vi "Repack Pixels_Pixel Bus to FIFO U1x8.vi"(10 "Input Valid":bool=TRUE, 11 "Pixel Bus In":T1={"Pixel Data"=[FALSE, FALSE, FALSE, FALSE, FALSE, FALSE, FALSE, FALSE], "DV"=[FALSE, FALSE, FALSE, FALSE, FALSE, FALSE, FALSE, FALSE], "EOL"=FALSE, "EOI"=FALSE, "Data Type"=enum."U1 x 8"}) -> (2 "Output Valid":bool, 3 "output array":bool[](array[boolean]))   [LabVIEW 2017, in "NI_VDM_FPGA_Basics.lvlib"]
uses:
  <vilib>/visionFPGA/NI_VDM_FPGA_Basics.lvlib
  <vilib>/visionFPGA/Controls/IMAQ FPGA Pixel Bus u1x8.ctl
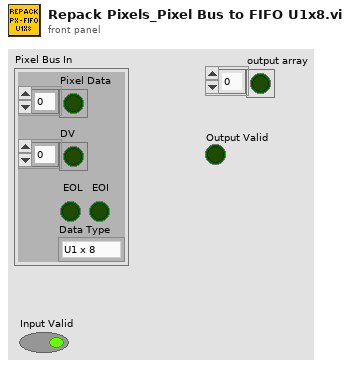
[diagram p1: front panel]
types:
  T1 = typedef "IMAQ FPGA Pixel Bus u1x8.ctl" = cluster{"Pixel Data":bool[], "DV":bool[], "EOL":bool, "EOI":bool, "Data Type":enum16{"U1 x 8"}}
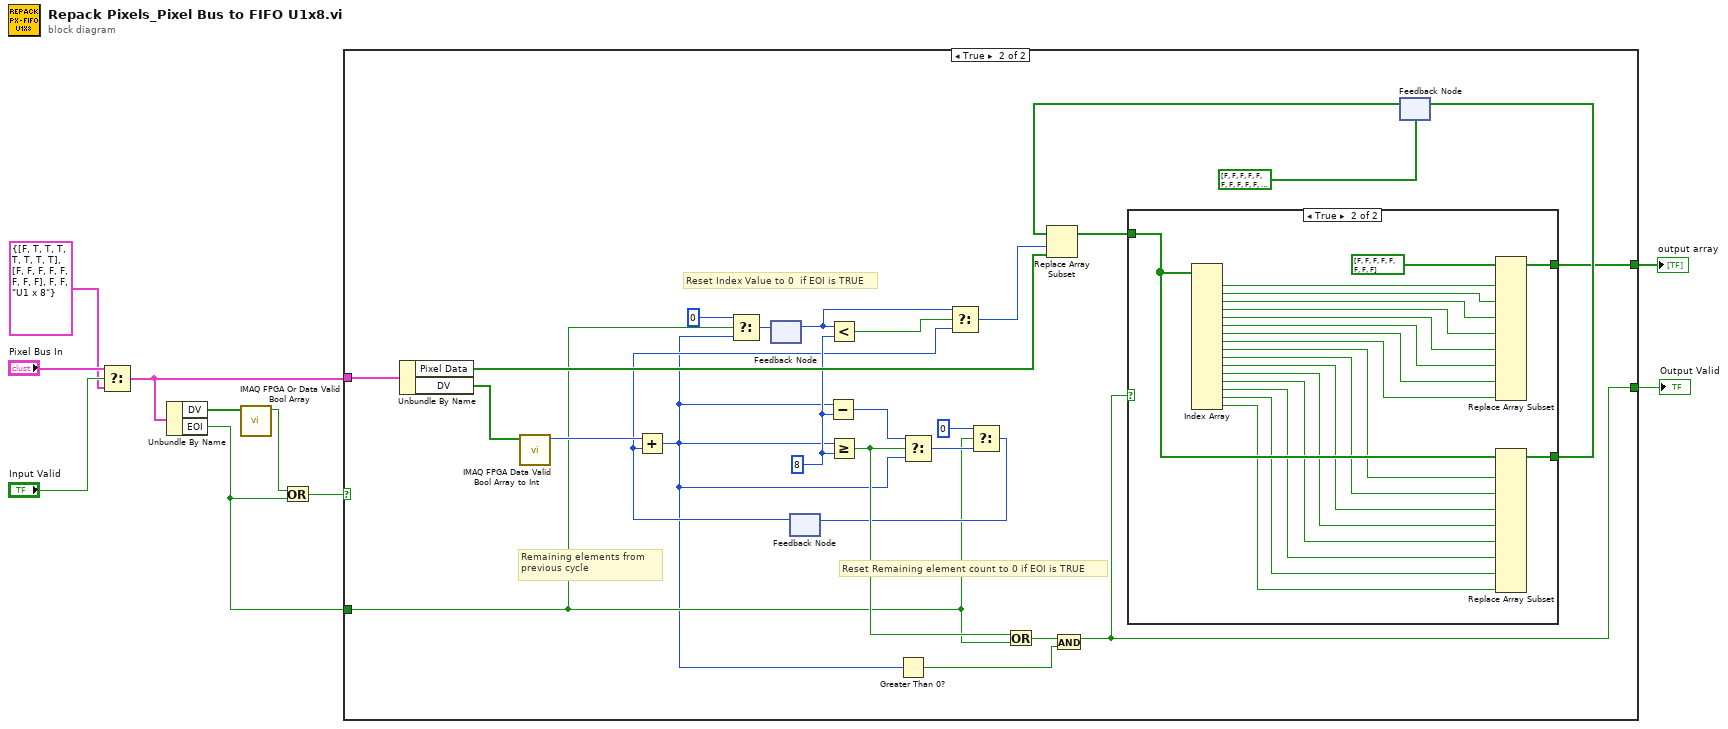
[diagram p0: block diagram]
diagram:
  n1 = Select(t="Pixel Bus In", s="Input Valid", f=T1 {"Pixel Data"=[FALSE, TRUE, TRUE, TRUE, TRUE, TRUE, TRUE, TRUE], "DV"=[FALSE, FALSE, FALSE, FALSE, FALSE, FALSE, FALSE, FALSE], "EOL"=FALSE, "EOI"=FALSE, "Data Type"=enum."U1 x 8"} ("Pixel Bus In")) -> (s? t:f=w6:T1)
  n2 = Unbundle By Name(w6) -> ("DV"=w5:bool[], "EOI"=w3:bool)
  n3 = call <vilib>:"IMAQ FPGA Or Data Valid Bool Array.vi"("DV Array In"=w5) -> ("DV Out"=w4:bool)  [unwired: 10 in]
  n4 = Or(x=w4, y=w3) -> (x .or. y?=w9:bool)
  n5 = case shown="True" w9 {
    tunnel: w6 -> [_ w36]
    tunnel: [_ w31] -> w1
    tunnel: [_ w14] -> w10
    tunnel: w3 -> [_ w15]
    frame False {
    }
    frame True {
      w29 = u16 8 ("y")
      # "Reset Remaining element count to 0 if EOI is TRUE"
      # "Reset Index Value to 0  if EOI is TRUE"
      # "Remaining elements from \nprevious cycle"
      n6 = Unbundle By Name(w36) -> ("Pixel Data"=w33:bool[], "DV"=w24:bool[])
      n7 = call <vilib>:"IMAQ FPGA Data Valid Bool Array to Int.vi"("DV In"=w24) -> ("Sum DV Out"=w23:u8)  [unwired: 10 in]
      n8 = feedback #1() -> (w28:u16)  [unwired: 1 in]
      n9 = feedback #2() -> (w22:u16)  [unwired: 1 in]
      n10 = Add(x=w23, y=w22) -> (x+y=w13:u16)
      n11 = Select(t=u16 0, s=w15, f=w13) -> (s? t:f=w17:u16)
      n12 = feedback-in #1(w17) -> ()
      n13 = Subtract(x=w13, y=w29) -> (x-y=w30:u16)
      n14 = Less?(x=w28, y=w29) -> (x < y?=w26:bool)
      n15 = Greater Or Equal?(x=w13, y=w29) -> (x >= y?=w25:bool)
      n16 = Greater Than 0?(x=w13) -> (x > 0?=w12:bool)
      n17 = Select(t=w30, s=w25, f=w13) -> (s? t:f=w20:u16)
      n18 = Select(t=w28, s=w26, f=w22) -> (s? t:f=w27:u16)
      n19 = Select(t=u16 0, s=w15, f=w20) -> (s? t:f=w18:u16)
      n20 = feedback-in #2(w18) -> ()
      n21 = Or(x=w25, y=w15) -> (x .or. y?=w21:bool)
      n22 = And(x=w21, y=w12) -> (x .and. y?=w14:bool)
      n23 = feedback #3(bool[] [FALSE, FALSE, FALSE, FALSE, FALSE, FALSE, FALSE, FALSE, FALSE, FALSE, FALSE, FALSE, FALSE, FALSE, FALSE, FALSE] ("Pixel Data")) -> (w34:bool[])
      n24 = Replace Array Subset(array=w34, new element=w33, index=w27) -> (w32:bool[])
      n25 = case shown="True" w14 {
        tunnel: [w37 w57] -> w35
        tunnel: w32 -> [w37 w56]
        tunnel: [_ w39] -> w31
        frame False {
        }
        frame True {
          n26 = Index Array(array=w56) -> (element #1=w55:bool, element #2=w54:bool, element #3=w53:bool, element #4=w52:bool, element #5=w51:bool, element #6=w50:bool, element #7=w49:bool, element #8=w48:bool, element #9=w47:bool, element #10=w46:bool, element #11=w45:bool, element #12=w44:bool, element #13=w43:bool, element #14=w42:bool, element #15=w41:bool, element #16=w40:bool)  [unwired: 16 in]
          n27 = Replace Array Subset(array=bool[] [FALSE, FALSE, FALSE, FALSE, FALSE, FALSE, FALSE, FALSE] ("Pixel Data"), new element #1=w55, new element #2=w54, new element #3=w53, new element #4=w52, new element #5=w51, new element #6=w50, new element #7=w49, new element #8=w48) -> (w39:bool[])  [unwired: 8 in]
          n28 = Replace Array Subset(array=w56, new element #1=w47, new element #2=w46, new element #3=w45, new element #4=w44, new element #5=w43, new element #6=w42, new element #7=w41, new element #8=w40) -> (w57:bool[])  [unwired: 8 in]
        }
      }
      n29 = feedback-in #3(w35) -> ()
    }
  }
  "output array" <- w1
  "Output Valid" <- w10
